vi "LED Spike Wrapper.vi"(1 "Camera LED ON/OFF":bool, 2 "Mode":enum8{"Start", "Run", "Finish"}(ring)) -> ()   [LabVIEW 2014]
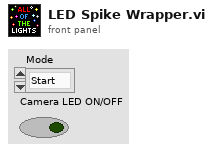
[diagram p1: front panel]
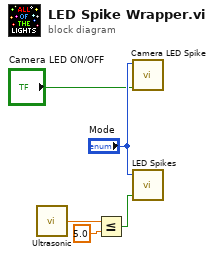
[diagram p0: block diagram]
diagram:
  n1 = call "Ultrasonic.vi"() -> ("Distance"=w5:dbl)  [unwired: 1 in]
  n2 = Less Or Equal?(x=w5, y=5.0) -> (x <= y?=w3:bool)
  n3 = call "Camera LED Spike.vi"("ON/OFF"="Camera LED ON/OFF", "Mode"="Mode") -> ()  [unwired: 10 in]
  n4 = call "LED Spikes.vi"("Light  2"=w3, "Mode"="Mode") -> ()  [unwired: 2 in]
